vi "kinematics (SubVI).vi"(6 "Bkt angle(deg)":sgl, 9 "Arm angle(deg)":sgl, 10 "Boom angle(deg)":sgl, 11 "Swing angle(deg)":sgl) -> (1 "beta_deg":dbl, 2 "alpha_deg":dbl, 3 "T":dbl[][](array[numeric]), 4 "gamma_deg":dbl)   [LabVIEW 2020]
uses:
  <vilib>/imath/engines/lvmath2/RunTimeEngine/IndexReplace/NIMS M(S,S)=S.vi
  <vilib>/imathl/engines/lvmath/Functions/Error Handling/Create Error.vi
  <vilib>/imath/engines/lvmath2/RunTimeEngine/NodeEndStatement/NIMS_NodeEndStatement_Output.vi
  <vilib>/imath/engines/lvmath2/RunTimeEngine/ErrorHandling/NIMS_Finalize Error.vi
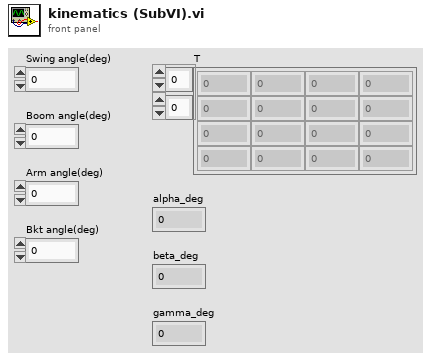
[diagram p1: front panel]
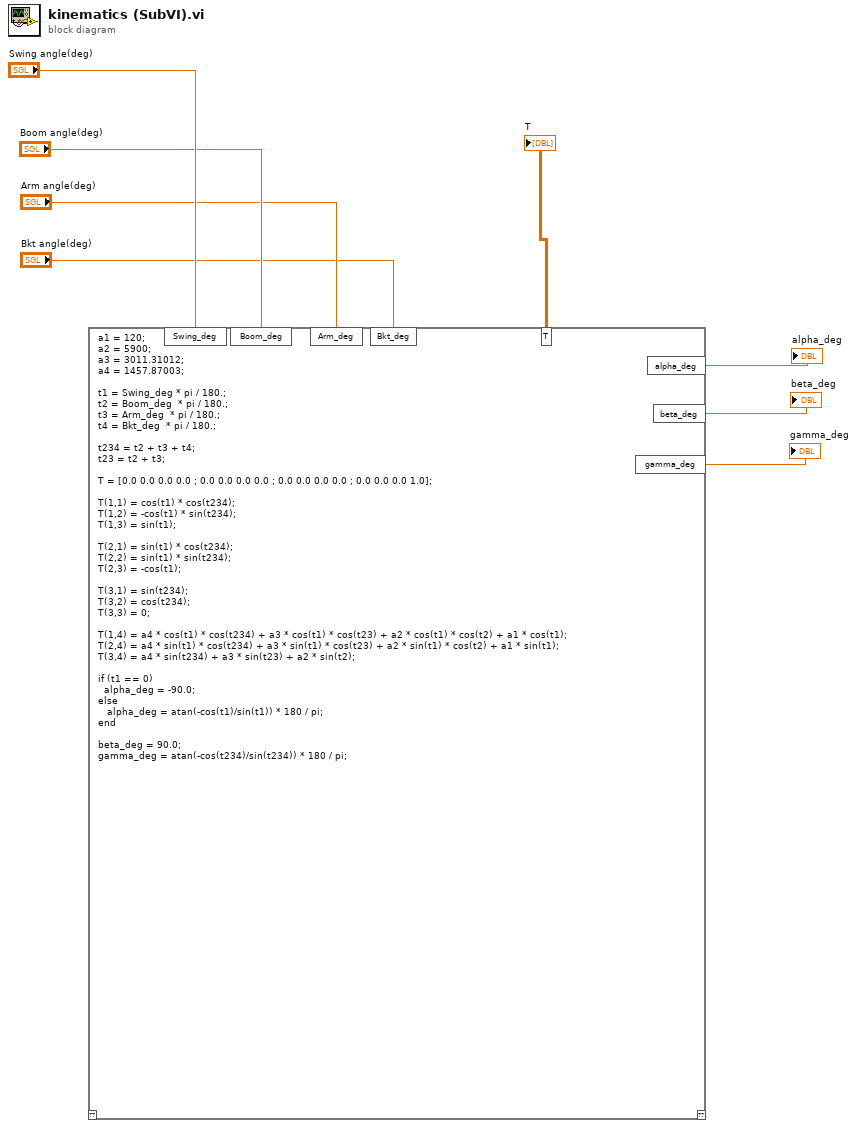
[diagram p0: block diagram]
diagram:
  n1 = mathscript code="a1 = 120;\na2 = 5900;\na3 = 3011.31012;\na4 = 1457.87003;\n\nt1 = Swing_deg * pi / 180.;\nt2 = Boom_deg  * pi / 180.;\nt3 = Arm_deg  * pi / 180.;\nt4 = Bkt_deg  * pi / 180.;\n\nt234 = t2 + t3 + t4;\nt23 = t2 + t3;\n\nT = [0.0 0.0 0.0 0.0 ; 0.0 0.0 0.0 0.0 ; 0.0 0.0 0.0 0.0 ; 0.0 0.0 0.0 1.0];\n\nT(1,1) = cos(t1) * cos(t234);\nT(1,2) = -cos(t1) * sin(t234);\nT(1,3) = sin(t1);\n\nT(2,1) = sin(t1) * cos(t234);\nT(2,2) = sin(t1) * sin(t234);\nT(2,3) = -cos(t1);\n\nT(3,1) = sin(t234);\nT(3,2) = cos(t234);\nT(3,3) = 0;\n\nT(1,4) = a4 * cos(t1) * cos(t234) + a3 * cos(t1) * cos(t23) + a2 * cos(t1) * cos(t2) + a1 * cos(t1);\nT(2,4) = a4 * sin(t1) * cos(t234) + a3 * sin(t1) * cos(t23) + a2 * sin(t1) * cos(t2) + a1 * sin(t1);\nT(3,4) = a4 * sin(t234) + a3 * sin(t23) + a2 * sin(t2);\n\nif (t1 == 0)\n  alpha_deg = -90.0;\nelse\n   alpha_deg = atan(-cos(t1)/sin(t1)) * 180 / pi;\nend\n\nbeta_deg = 90.0;\ngamma_deg = atan(-cos(t234)/sin(t234)) * 180 / pi;"("Swing_deg"="Swing angle(deg)", "Boom_deg"="Boom angle(deg)", "Arm_deg"="Arm angle(deg)", "Bkt_deg"="Bkt angle(deg)") -> ("T"=→"T":dbl[][], "alpha_deg"=→"alpha_deg":cdb, "beta_deg"=→"beta_deg":dbl, "gamma_deg"=→"gamma_deg":cdb)  [unwired: 1 in, 1 out]
